vi "Process.vi"(8 "error in":errorcluster, 11 "Instrument":refnum<class "Instrument.lvclass">) -> (0 "error out":errorcluster, 3 "Instrument out":refnum<class "Instrument.lvclass">)   [LabVIEW 2019, in "Instrument.lvclass"]
doc: "---------------------------------------------------------------\nJKI State Machine Objects™\nhttp://jki.net/state-machine-objects/\nCopyright (C) 2005-2015, JKI <info@jki.net>\nALL RIGHTS RESERVED"
uses:
  Instrument.lvclass
  C:/Program Files (x86)/National Instruments/LabVIEW 2019/vi.lib/JKI/JKI SMO/SMO/SMO.lvclass
  Typedefs/PrivateEvents--Instrument.DataToLog.ctl
  Instrument.lvclass/Instrument.ctl
  <userlib>/LevyLab/RemoteControl/Typedefs/Message--Cluster.ctl
  Typedefs/PrivateEvents--LogTime.ctl
  <vilib>/JKI/JKI SMO/SMO/SMO.lvclass/SMO.ctl
  <vilib>/JKI/JKI SMO/SMO/Private/ReftoDVR--SMO.vi
  <userlib>/LevyLab/RemoteControl/RemoteControl.lvclass
  <userlib>/LevyLab/Logger.Error/Logger.Error.lvclass
  <userlib>/LevyLab/Logger.PGSQL/Logger.PGSQL.lvclass
  <vilib>/JKI/JKI SMO/SMO/SMO.lvclass
  C:/Program Files (x86)/National Instruments/LabVIEW 2019/user.lib/LevyLab/Logger/Logger.lvclass
  <userlib>/LevyLab/Configuration/Debug.lvlib
panel:
  out "State History":string
  out "Name":string
  out "Command":string
  # "1. Receives & processes commands from RemoteControl process\n2. Logs instrument settings to PGSQL using Logger process"
  # "INSTRUMENT"
  # "INSTRUMENT"
  # "For instructions on how to use the JKI State Machine Objects, examples and video tutorials, visit:\nhttp://jki.net/state-machine-objects/\n\nJKI State Machine Objects™\nhttp://jki.net/state-machine-objects/\nCopyright (C) 2005-2015, JKI <info@jki.net>\nALL RIGHTS RESERVED"
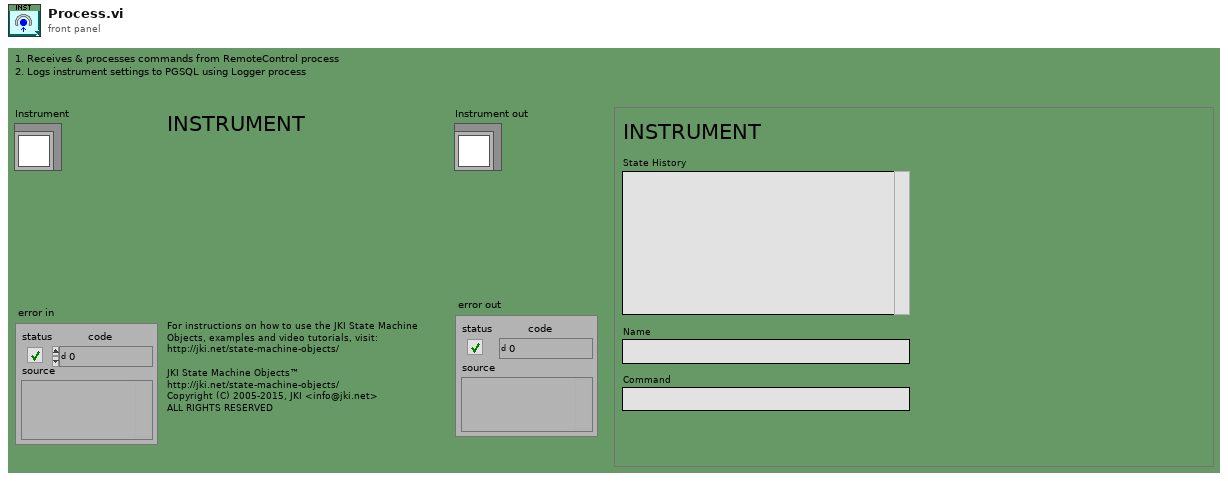
[diagram p1: front panel]
types:
  T1 = typedef "Instrument.lvclass/PrivateEvents--Instrument.DataToLog.ctl" = cluster{"path":string, "Data":variant}
  T2 = enum32{"invalid app kind", "Development System", "Run Time System", "Student Edition", "Embedded LabVIEW", "Evaluation", "Custom"}
  T3 = enum32{"Invalid", "Standard", "Closed", "Hidden", "Minimized", "Maximized"}
  T4 = typedef "RemoteControl.lvclass/Message--Cluster.ctl" = cluster{"Command":string, "Data":variant, "ID":string}
  T5 = typedef "Instrument.lvclass/PrivateEvents--LogTime.ctl" = u32
  T6 = typedef "Instrument.lvclass/Dependencies--Cluster.ctl" = cluster{"API":refnum<class "API.lvclass">, "Configuration":refnum<class "Configuration.lvclass">, "HAL":refnum<class "HAL.lvclass">, "DB-Logger":refnum<class "Logger.PGSQL.lvclass">, "Error-Logger":refnum<class "Logger.Error.lvclass">, "Remote-Control":refnum<class "RemoteControl.lvclass">}
  T7 = typedef "Debug.lvlib/Attribute.Debug.lvclass/DebugBehavior.ctl" = enum16{"Normal", "Debug"}
  T8 = cluster{"Core":cluster{"Current VI Reference":refnum<vi>, "Close Panel on Exit?":bool, "Last Error":cluster{"error":errorcluster, "previous state":string, "remaining states":string}, "Shutdown?":bool}, "SelfRef":refnum<class "Instrument.lvclass">, "Dependencies":T6, "Message":T4, "LogTime":T5, "Behavior":T7}
  T9 = typedef "SMO.lvclass/SMOState --Enum.ctl" = enum16{"unknown", "Created", "Started", "Stopped"}
  T10 = cluster{"Current VI Reference":refnum<vi>, "Close Panel on Exit?":bool, "Last Error":cluster{"error":errorcluster, "previous state":string, "remaining states":string}, "Shutdown?":bool}
  T11 = typedef "SMO.lvclass/Protected Events.ctl" = cluster{"StopProcesses":refnum<user-event>, "AbortProcesses":refnum<user-event>, "Config Changed":refnum<user-event>, "Dependency":refnum<user-event>}
  T12 = typedef "Instrument.lvclass/PrivateEvents--Cluster.ctl" = cluster{"MessageToProcess":refnum<user-event>, "LogData":refnum<user-event>, "LogTime":refnum<user-event>}
  T13 = typedef "RemoteControl.lvclass/PublicEvents--Cluster.ctl" = cluster{"SendMessageFromProcess":refnum<user-event>}
  T14 = typedef "SMO.lvclass/Public Events.ctl" = cluster{"Error":refnum<user-event>, "State":refnum<user-event>, "Reserve State":refnum<user-event>}
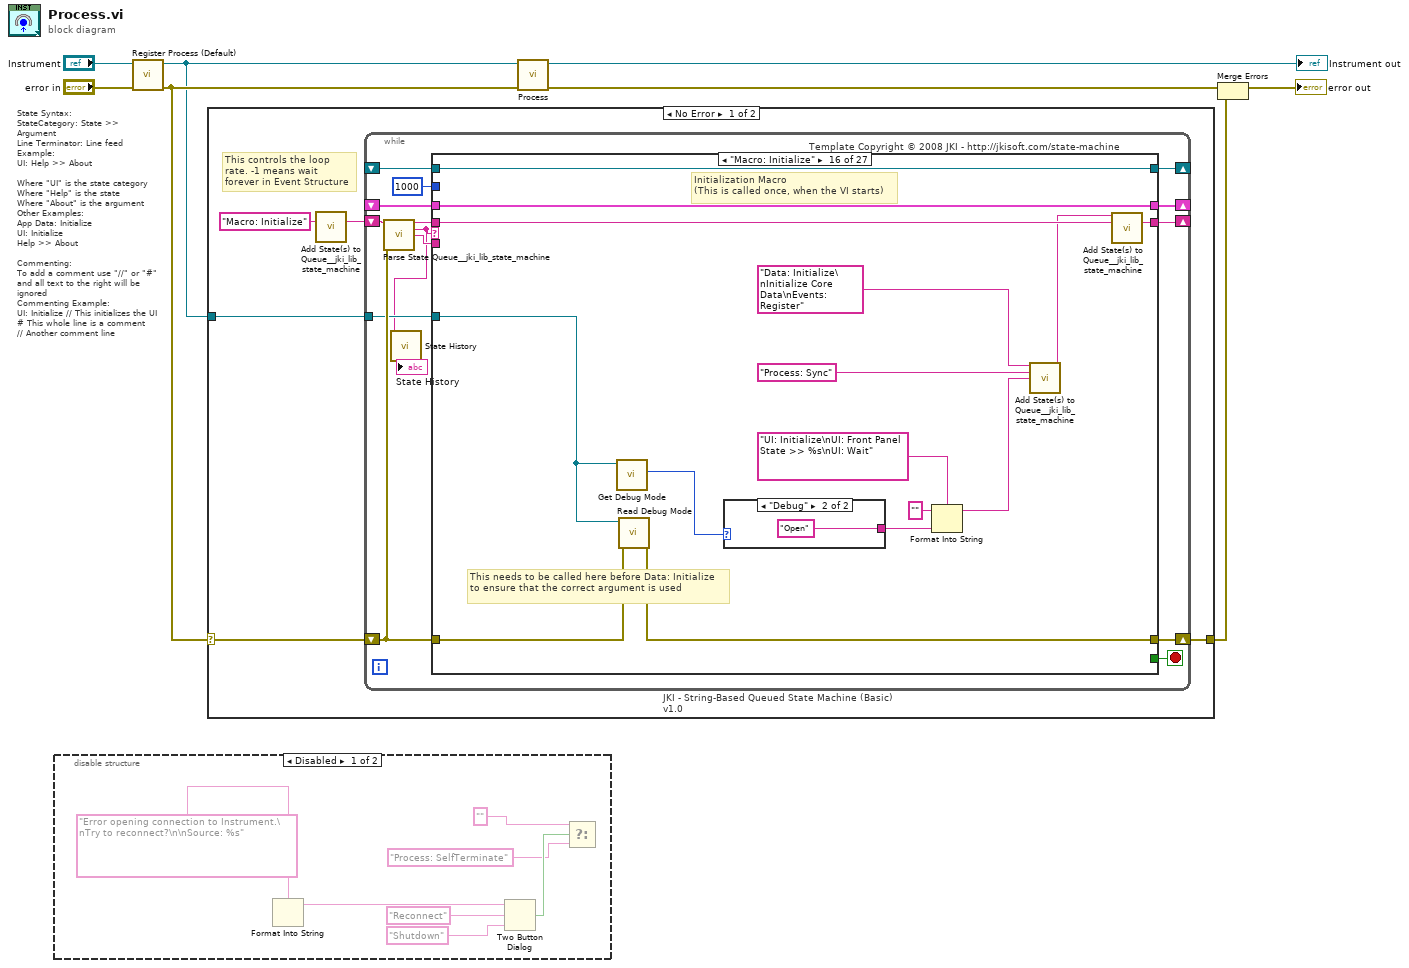
[diagram p0: block diagram]
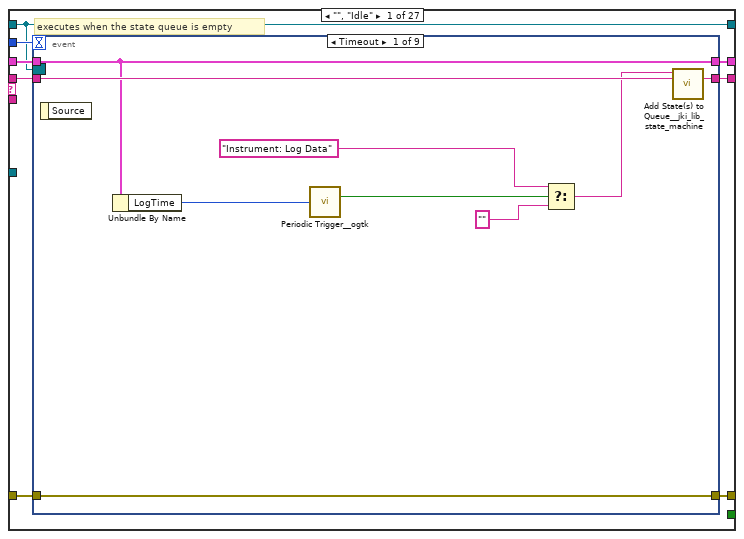
[diagram p3: hidden frame]
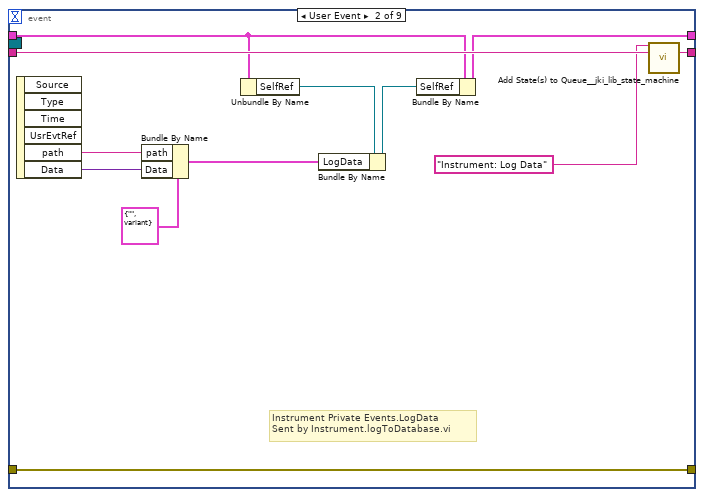
[diagram p4: hidden frame]
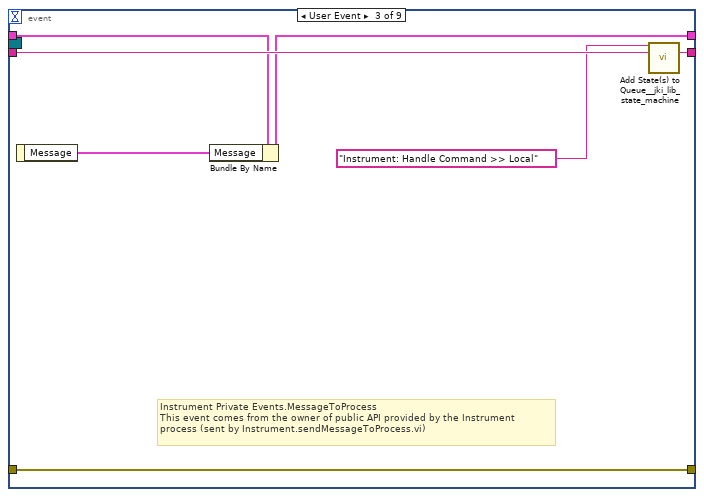
[diagram p5: hidden frame]
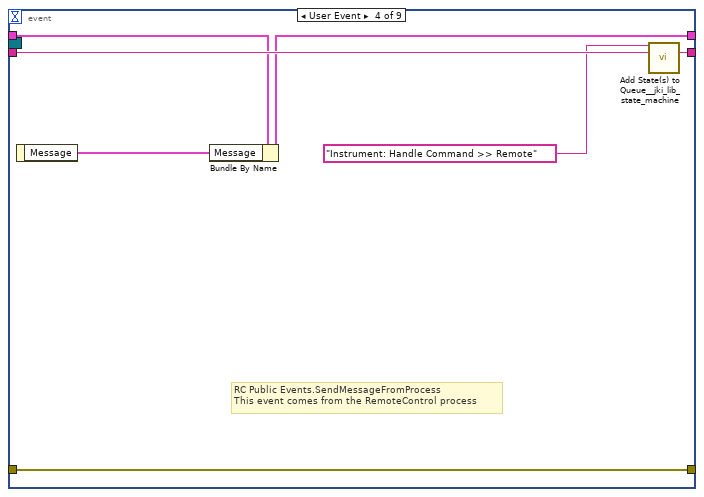
[diagram p6: hidden frame]
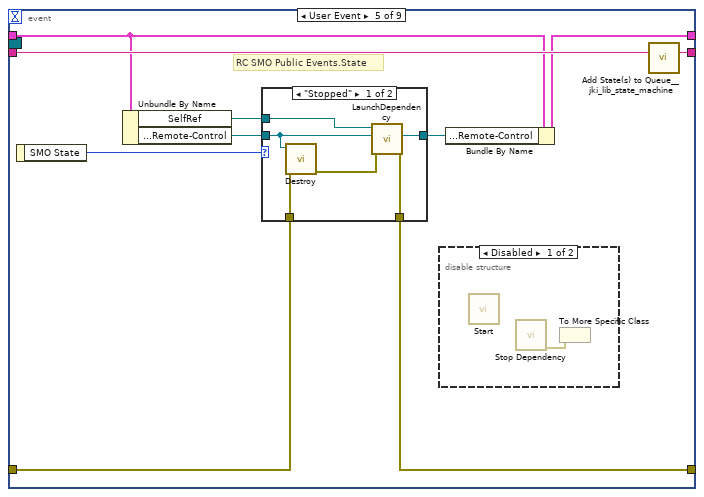
[diagram p7: hidden frame]
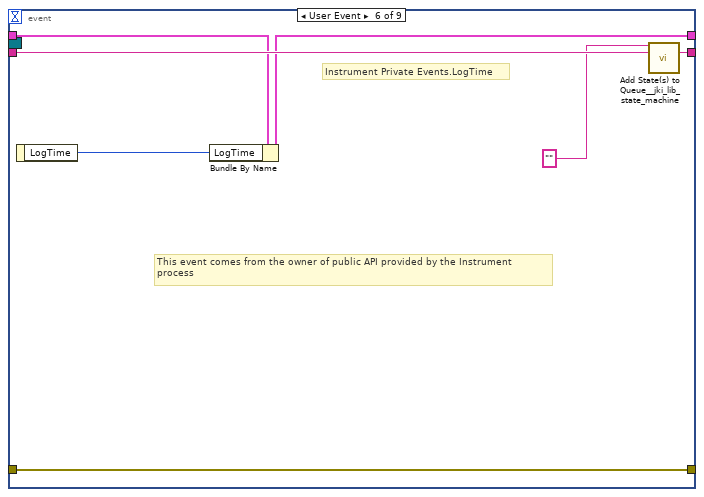
[diagram p10: hidden frame]
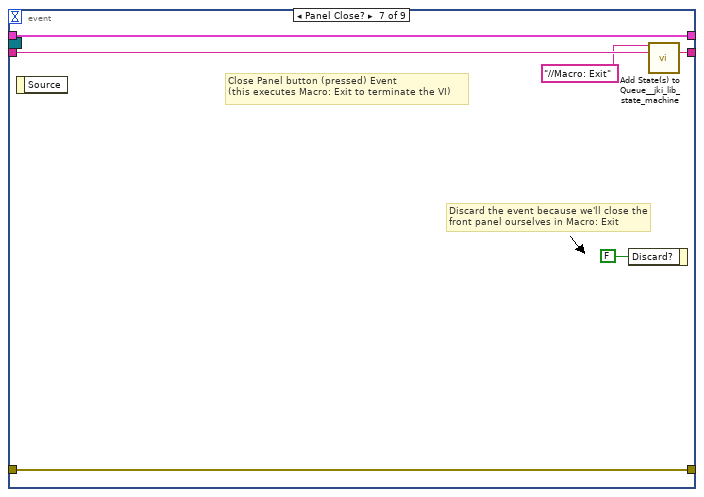
[diagram p11: hidden frame]
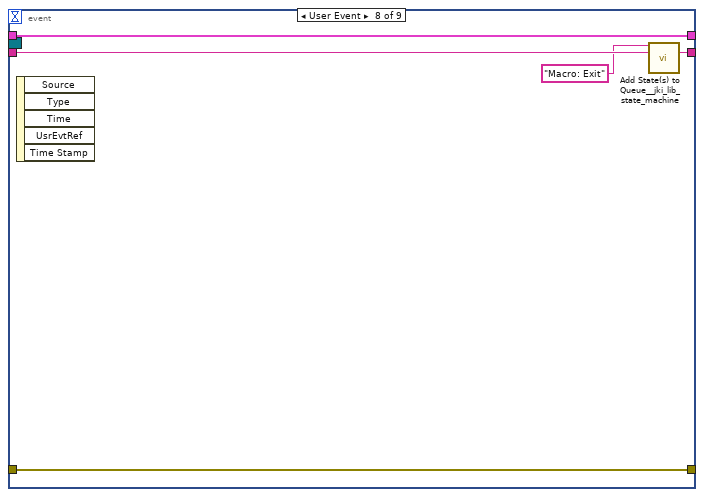
[diagram p12: hidden frame]
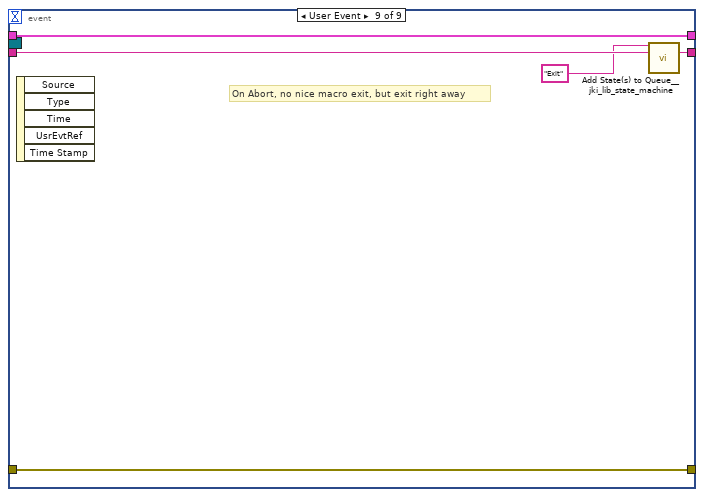
[diagram p13: hidden frame]
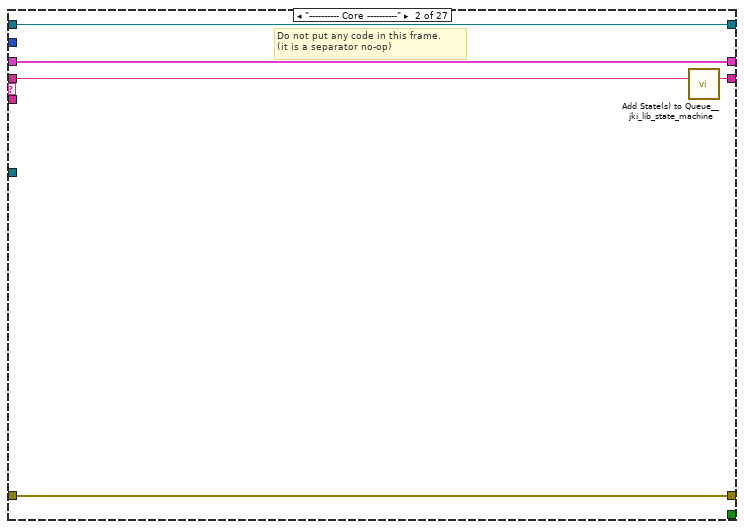
[diagram p14: hidden frame]
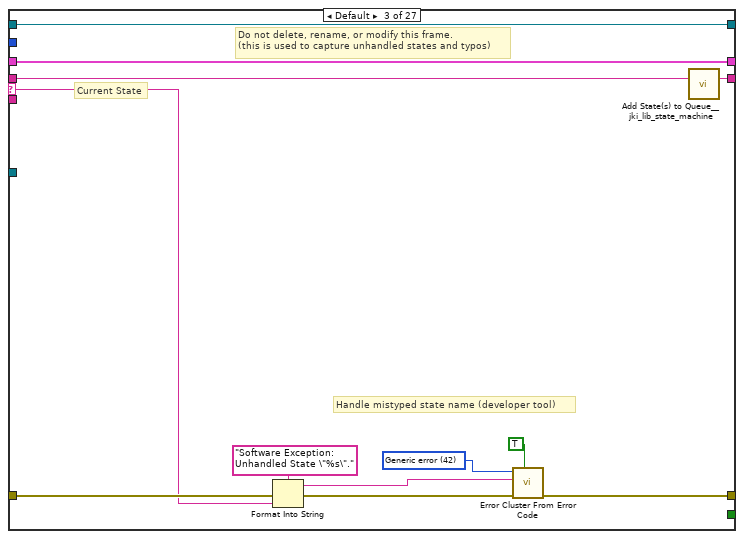
[diagram p15: hidden frame]
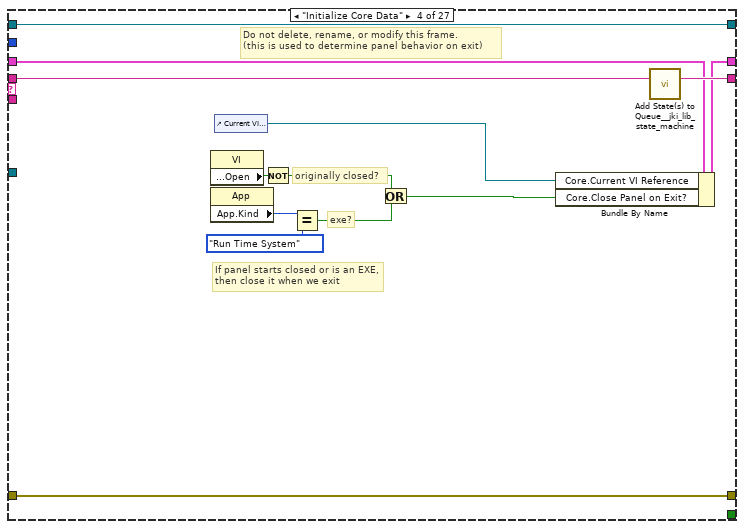
[diagram p16: hidden frame]
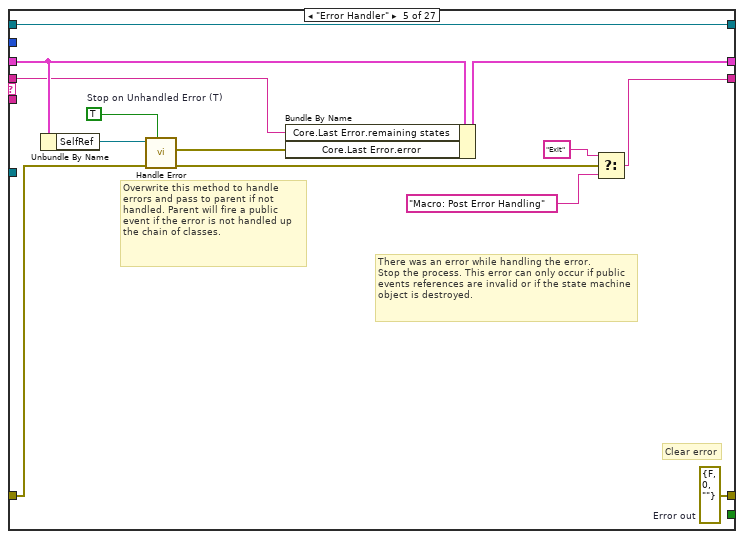
[diagram p17: hidden frame]
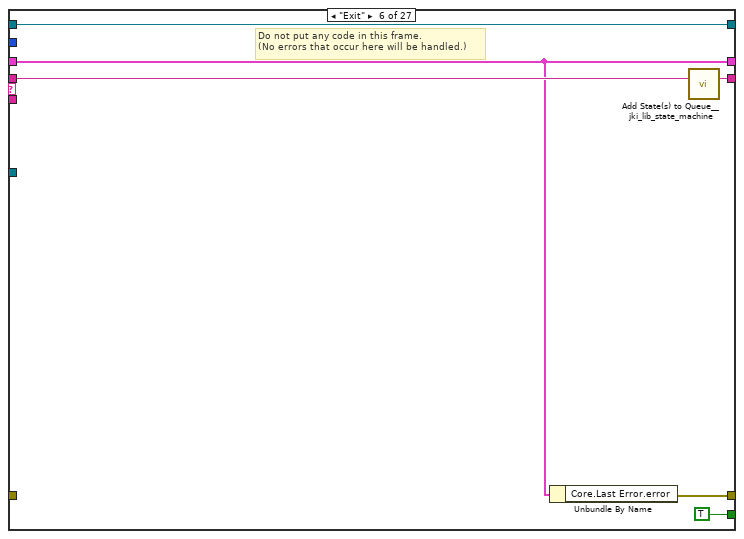
[diagram p18: hidden frame]
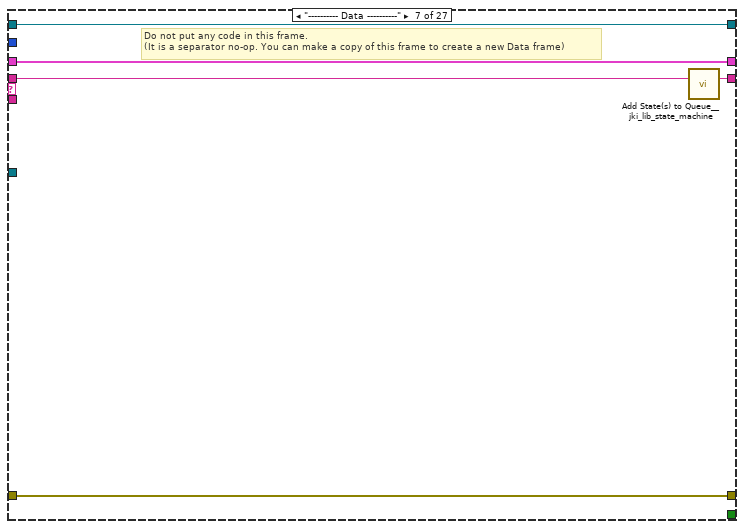
[diagram p19: hidden frame]
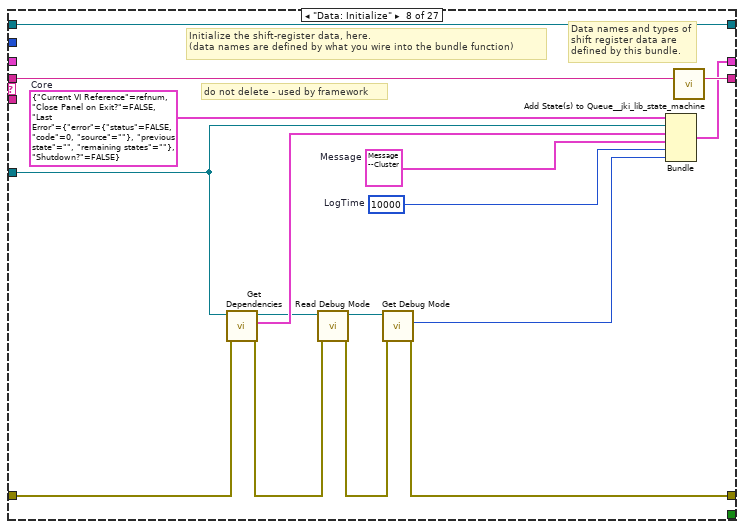
[diagram p20: hidden frame]
diagram:
  # "State Syntax:\nStateCategory: State >> Argument\nLine Terminator: Line feed\nExample:\nUI: Help >> About\n\nWhere \"UI\" is the state category\nWhere \"Help\" is the state\nWhere \"About\" is the argument\nOther Examples:\nApp Data: Initialize\nUI: Initialize\nHelp >> About\n\nCommenting:\nTo add a comment use \"//\" or \"#\" and all text to the right will be ignored\nCommenting Example:\nUI: Initialize // This initializes the UI\n# This whole line is a comment\n// Another comment line"
  n1 = disable-structure shown="Disabled" {
    frame Disabled {
      n2 = Format Into String(format string="Error opening connection to Instrument.\nTry to reconnect?\n\nSource: %s" ("message")) -> (resulting string=w9:string)  [unwired: 3 in, 1 out]
      n3 = Two Button Dialog(message=w9, 1:"Shutdown" ("F button name (\"Cancel\")"), 2:"Reconnect" ("T button name (\"OK\")")) -> (T button?=w13:bool)
      n4 = Select(t="" ("States to Execute"), s=w13, f="Process: SelfTerminate" ("States to Execute")) -> ()  [unwired: 1 out]
    }
    frame Enabled {
    }
  }
  n5 = call <vilib>:"Register Process (Default).vi"("error in (no error)"="error in", "SMO"="Instrument") -> ("error out"=w5:errorcluster, "SelfRef"=w4:refnum<class "Instrument.lvclass">)  [unwired: 8 in]
  n6 = case shown="No Error" w5 {
    selector: w5 -> [w17 w462]
    tunnel: w4 -> [w18 _]
    tunnel: [w16 w462] -> w1
    frame No Error {
      # "This controls the loop rate. -1 means wait forever in Event Structure"
      n7 = call <vilib>:"Add State(s) to Queue__jki_lib_state_machine.vi"("State(s) in (\"\")"="Macro: Initialize") -> ("States Out"=w20:string)  [unwired: 14 in]
      n8 = while "JKI - String-Based Queued State Machine (Basic) v1.0" {
        shift-right: [w29] -> _
        shift-left: _ -> [w28]
        shift-right: [w32] -> w16
        shift-left: w17 -> [w26]
        shift-right: [w31] -> _
        shift-left: w20 -> [w33]
        tunnel: w18 -> [w23]
        shift-right: [w25] -> _
        shift-left: _ -> [w24]
        stop <- w30 stop-if-true
        # "Template Copyright © 2008 JKI - http://jkisoft.com/state-machine"
        n9 = call <vilib>:"Parse State Queue__jki_lib_state_machine.vi"("State Queue"=w33, "Error In (no error)"=w26) -> ("Remaining States"=w35:string, "Current State"=w22:string, "Arguments"=w34:string)  [unwired: 11 in]
        n10 = call "State History.vi"("Current State"=w22) -> ("History"=→"State History":string)  [unwired: 10 in]
        n11 = case shown="\"Macro: Initialize\"" w22 {
          selector: w22 -> [_ _ w127 _ _ _ _ _ _ _ _ _ _ _ _ _ _ _ _ _ _ _ _ _ _ _ _]
          tunnel: w35 -> [w43 w125 w131 w150 w152 w169 w174 w190 w197 w202 w212 w219 w235 w270 w277 w292 w311 w317 w334 w345 w354 w359 w390 w396 w401 w424 w461]
          tunnel: w34 -> [_ _ _ _ _ _ _ _ _ _ _ w213 w229 _ _ _ _ _ _ _ _ _ _ _ _ w404 _]
          tunnel: w28 -> [w41 w122 w129 w141 w161 w165 w171 _ w192 w199 w209 w217 w231 w265 w274 w286 w303 w320 w331 w342 w349 w356 w388 w394 w399 w417 w455]
          tunnel: [w40 w123 w133 w147 w162 w164 w172 w175 w193 w200 w203 w214 w232 w266 w275 w284 w309 w324 w332 w336 w346 w357 w386 w392 w397 w409 w456] -> w32
          tunnel: w26 -> [w39 w123 w132 w147 w153 _ w172 w180 w194 w200 w206 w215 w233 w267 w275 w285 w309 w324 w332 w337 w347 w357 w384 w392 w397 w420 w457]
          tunnel: [w42 w124 w130 w149 w157 w168 w173 w189 w196 w201 w211 w218 w234 w269 w276 w291 w310 w318 w333 w344 w353 w358 w389 w395 w400 w423 w460] -> w31
          tunnel: [_ _ _ _ _ TRUE _ _ _ _ _ _ _ _ _ _ _ _ _ _ _ _ _ _ _ _ _] -> w30
          tunnel: [w38 w122 w129 w148 w160 w165 w171 w184 w192 w199 w209 w217 w231 w265 w274 w286 w303 w321 w331 w342 w348 w356 w388 w394 w399 w416 w455] -> w29
          tunnel: 1000 ("Timeout") -> [w37 _ _ _ _ _ _ _ _ _ _ _ _ _ _ _ _ _ _ _ _ _ _ _ _ _ _]
          tunnel: [w36 w121 w126 w138 w163 w166 w170 w188 w191 w198 w210 w216 w228 w268 w273 w290 w304 w325 w330 w343 w352 w355 w387 w393 w398 w422 w459] -> w25
          tunnel: w24 -> [w36 w121 w126 w138 w163 w166 w170 w188 w191 w198 w210 w216 w228 w268 w273 w290 w304 w325 w330 w343 w352 w355 _ w393 w398 w422 w459]
          tunnel: w23 -> [_ _ _ _ _ _ _ w182 _ _ _ _ _ _ _ w280 _ _ _ _ _ _ _ _ _ _ _]
          frame "", "Idle" {
            # "executes when the state queue is empty"
            n12 = event shown="[0] Timeout" {
              selector: w36 -> [_ _ _ _ _ _ _ _ _]
              dyn-events: _ -> [_ _ _ _ _ _ _ _ _]
              timeout: w37 -> [_ _ _ _ _ _ _ _ _]
              tunnel: w43 -> [w52 w64 w71 w78 w88 w104 w110 w115 w120]
              tunnel: [w51 w63 w70 w77 w87 w103 w109 w114 w119] -> w42
              tunnel: w41 -> [w45 w55 w68 w75 w84 w101 w107 w112 w117]
              tunnel: [w50 w62 w69 w76 w81 w102 w108 w113 w118] -> w40
              tunnel: w39 -> [w50 w62 w69 w76 w82 w102 w108 w113 w118]
              tunnel: [w45 w53 w67 w74 w83 w100 w107 w112 w117] -> w38
              event Timeout {
                n13 = event-data() -> ()  [unwired: 1 in, 1 out]
                n14 = Unbundle By Name(w45) -> ("LogTime"=w44:T5)
                n15 = call <userlib>:"Periodic Trigger__ogtk.vi"("time (ms)"=w44) -> ("Triggered"=w48:bool)  [unwired: 12 in, 2 out]
                n16 = Select(t="Instrument: Log Data" ("State(s) in Front (\"\")"), s=w48, f="") -> (s? t:f=w49:string)
                n17 = call <vilib>:"Add State(s) to Queue__jki_lib_state_machine.vi"("State(s) in Front (\"\")"=w49, "State(s) in (\"\")"=w52) -> ("States Out"=w51:string)  [unwired: 13 in]
              }
              event User Event {
                # "Instrument Private Events.LogData\nSent by Instrument.logToDatabase.vi"
                n18 = event-data() -> ("path"=w58:string, "Data"=w59:variant)  [unwired: 1 in, 4 out]
                n19 = Bundle By Name(cluster=T1 {"path"="", "Data"=variant} ("Log Data"), "path"=w58, "Data"=w59) -> (w57:T1)
                n20 = Unbundle By Name(w55) -> ("SelfRef"=w56:refnum<class "Instrument.lvclass">)
                n21 = Bundle By Name(cluster=w56, "LogData"=w57) -> (w54:refnum<class "Instrument.lvclass">)
                n22 = Bundle By Name(cluster=w55, "SelfRef"=w54) -> (w53:T8)
                n23 = call <vilib>:"Add State(s) to Queue__jki_lib_state_machine.vi"("State(s) in Front (\"\")"="Instrument: Log Data" ("State(s) in Front (\"\")"), "State(s) in (\"\")"=w64) -> ("States Out"=w63:string)  [unwired: 13 in]
              }
              event User Event {
                # "Instrument Private Events.MessageToProcess\nThis event comes from the owner of public API provided by the Instrument\nprocess (sent by Instrument.sendMessageToProcess.vi)"
                n24 = event-data() -> ("Message"=w66:T4)  [unwired: 1 in]
                n25 = Bundle By Name(cluster=w68, "Message"=w66) -> (w67:T8)
                n26 = call <vilib>:"Add State(s) to Queue__jki_lib_state_machine.vi"("State(s) in Front (\"\")"="Instrument: Handle Command >> Local" ("State(s) in Front (\"\")"), "State(s) in (\"\")"=w71) -> ("States Out"=w70:string)  [unwired: 13 in]
              }
              event User Event {
                # "RC Public Events.SendMessageFromProcess\nThis event comes from the RemoteControl process"
                n27 = event-data() -> ("Message"=w73:T4)  [unwired: 1 in]
                n28 = Bundle By Name(cluster=w75, "Message"=w73) -> (w74:T8)
                n29 = call <vilib>:"Add State(s) to Queue__jki_lib_state_machine.vi"("State(s) in Front (\"\")"="Instrument: Handle Command >> Remote" ("State(s) in Front (\"\")"), "State(s) in (\"\")"=w78) -> ("States Out"=w77:string)  [unwired: 13 in]
              }
              event User Event {
                # "RC SMO Public Events.State"
                n30 = event-data() -> ("SMO State"=w79:T9)  [unwired: 1 in]
                n31 = Unbundle By Name(w84) -> ("SelfRef"=w80:refnum<class "Instrument.lvclass">, "Dependencies.Remote-Control"=w86:refnum<class "RemoteControl.lvclass">)
                n32 = case shown="\"Stopped\"" w79 {
                  tunnel: w86 -> [w90 w97]
                  tunnel: [w95 w97] -> w85
                  tunnel: w82 -> [w92 w96]
                  tunnel: [w94 w96] -> w81
                  tunnel: w80 -> [w93 _]
                  frame "Stopped" {
                    n33 = call <vilib>:"Destroy.vi"("error in (no error)"=w92, "SMO"=w90) -> ("error out"=w91:errorcluster)  [unwired: 9 in]
                    n34 = call <vilib>:"LaunchDependency.vi"("error in (no error)"=w91, "Dependency Type"=w90, "SMO in"=w93) -> ("error out"=w94:errorcluster, "Dependency Reference"=w95:refnum<class "RemoteControl.lvclass">)  [unwired: 5 in, 2 out]
                  }
                  frame Default {
                  }
                }
                n35 = disable-structure shown="Disabled" {
                  frame Disabled {
                    n36 = call <vilib>:"Start.vi"() -> ()  [unwired: 10 in, 2 out]
                    n37 = call <vilib>:"Stop Dependency.vi"() -> ("error out"=w89:errorcluster)  [unwired: 9 in, 2 out]
                    n38 = To More Specific Class(error in=w89) -> ()  [unwired: 2 in, 2 out]
                  }
                  frame Enabled {
                  }
                }
                n39 = Bundle By Name(cluster=w84, "Dependencies.Remote-Control"=w85) -> (w83:T8)
                n40 = call <vilib>:"Add State(s) to Queue__jki_lib_state_machine.vi"("State(s) in (\"\")"=w88) -> ("States Out"=w87:string)  [unwired: 14 in]
              }
              event User Event {
                # "Instrument Private Events.LogTime"
                # "This event comes from the owner of public API provided by the Instrument\nprocess"
                n41 = event-data() -> ("LogTime"=w99:T5)  [unwired: 1 in]
                n42 = Bundle By Name(cluster=w101, "LogTime"=w99) -> (w100:T8)
                n43 = call <vilib>:"Add State(s) to Queue__jki_lib_state_machine.vi"("State(s) in Front (\"\")"="" ("State(s) in Front (\"\")"), "State(s) in (\"\")"=w104) -> ("States Out"=w103:string)  [unwired: 13 in]
              }
              event Panel Close? {
                # "Discard the event because we'll close the front panel ourselves in Macro: Exit"
                # "Close Panel button (pressed) Event\n(this executes Macro: Exit to terminate the VI)"
                n44 = event-data() -> ()  [unwired: 1 in, 1 out]
                n45 = event-data("Discard?"=FALSE) -> ()  [unwired: 1 in, 1 out]
                n46 = call <vilib>:"Add State(s) to Queue__jki_lib_state_machine.vi"("State(s) in Front (\"\")"="//Macro: Exit", "State(s) in (\"\")"=w110) -> ("States Out"=w109:string)  [unwired: 13 in]
              }
              event User Event {
                n47 = event-data() -> ()  [unwired: 1 in, 5 out]
                n48 = call <vilib>:"Add State(s) to Queue__jki_lib_state_machine.vi"("State(s) in Front (\"\")"="Macro: Exit", "State(s) in (\"\")"=w115) -> ("States Out"=w114:string)  [unwired: 13 in]
              }
              event User Event {
                # "On Abort, no nice macro exit, but exit right away"
                n49 = event-data() -> ()  [unwired: 1 in, 5 out]
                n50 = call <vilib>:"Add State(s) to Queue__jki_lib_state_machine.vi"("State(s) in Front (\"\")"="Exit", "State(s) in (\"\")"=w120) -> ("States Out"=w119:string)  [unwired: 13 in]
              }
            }
          }
          frame "---------- Core ----------" {
            # "Do not put any code in this frame.\n(it is a separator no-op)"
            n51 = call <vilib>:"Add State(s) to Queue__jki_lib_state_machine.vi"("State(s) in (\"\")"=w125) -> ("States Out"=w124:string)  [unwired: 14 in]
          }
          frame Default {
            w136 = 42 items=["No error", "Argument error", "Memory is full", "Out of zone", "End of file", "File already open", "Generic file I/O error", "File not found", "File permission error", "Disk is full", "Duplicate path", "Too many files open", "System feature not enabled", "Resource file not found", "Cannot add resource", "Resource not found", "Image not found", "Image memory error", "Pen does not exist", "Config type invalid", "Config token not found", "Config parse error", "Config memory error", "Bad external code format", "Bad external code offset", "External code not present", "Null window", "Destroy window error", "Null menu", "Print aborted", "Bad print record", "Print driver error", "Windows error during printing", "Memory error during printing", "Print dialog error", "Generic print error", "Invalid device refnum", "Device not found", "Device parameter error", "Device unit error", "Cannot open device", "Device call aborted", "Generic error", "Cancelled by user", "Object ID too low", "Object ID too high", "Object not in heap", "Unknown heap", "Unknown object (invalid DefProc)", "Unknown object (DefProc not in table)", "Message out of range", "Invalid (null) method", "Unknown message", "Manager call not supported", "Bad address", "Network operation in progress", "Network operation timed out", "Connection is busy", "Network attribute not supported", "Network error", "Address in use", "System out of memory", "Connection aborted", "Connection refused", "Not connected", "Already connected", "Connection closed", "Initialization error (interapplication manager)", "Bad occurrence", "Wait on unbound occurrence handler", "Occurrence queue overflow", "Datalog type conflict", "Unused", "Unrecognized type (interapplication manager)", "Memory corrupt", "Failed to make temporary DLL", "Old CIN version", "Drag socket not found", "Failed to load drop-object", "Failed to register OLE object", "Failed to release OLE object", "Format specifier type mismatch", "Unknown format specifier", "Too few format specifiers", "Too many format specifiers", "Scan failed", "Newer CIN version", "Error converting to variant", "Runtime menu error", "Password tampered", "Variant attribute not found", "Incompatible variant data type", "Event data is not available", "Event Store is not present", "Occurrence is not found", "Event Queue is not created", "Event info is not available", "Refnum passed is NULL", "Error retrieving Class GUID", "Error retrieving CoClass GUID", "Error retrieving TypeLib GUID.", "Bad built application magic bytes.", "Specific driver is different from the specific driver associated with the Logical Name.", "There is no session opened to the class driver.", "Max Error", "MAX - Error with config objects", "MAX - Error loading configuration", "MAX - Group not supported"]
            # "Current State"
            # "Do not delete, rename, or modify this frame.\n(this is used to capture unhandled states and typos)"
            # "Handle mistyped state name (developer tool)"
            n52 = Format Into String(format string="Software Exception: Unhandled State \"%s\"." ("message"), error in=w132, w127) -> (resulting string=w135:string, error out=w134:errorcluster)  [unwired: 1 in]
            n53 = call <vilib>:"Error Cluster From Error Code.vi"("show call chain? (False)"=TRUE, "error in (no error)"=w134, "error message (\"\")"=w135, "error code (0)"=w136) -> ("error out"=w133:errorcluster)  [unwired: 5 in]
            n54 = call <vilib>:"Add State(s) to Queue__jki_lib_state_machine.vi"("State(s) in (\"\")"=w131) -> ("States Out"=w130:string)  [unwired: 14 in]
          }
          frame "Initialize Core Data" {
            # "Do not delete, rename, or modify this frame.\n(this is used to determine panel behavior on exit)"
            # "originally closed?"
            # "exe?"
            # "If panel starts closed or is an EXE, then close it when we exit"
            n55 = property class="VI"() -> ("Front Panel.Open"=w146:bool)  [unwired: 2 in, 2 out]
            n56 = property class="App"() -> ("App.Kind"=w145:T2)  [unwired: 2 in, 2 out]
            n57 = control-ref of="Current VI Reference"() -> (w139:refnum<vi>)
            n58 = Not(x=w146) -> (.not. x?=w143:bool)
            n59 = Equal?(x=w145, y=T2."Run Time System" ("Application:Kind")) -> (x = y?=w142:bool)
            n60 = Or(x=w143, y=w142) -> (x .or. y?=w140:bool)
            n61 = Bundle By Name(cluster=w141, "Core.Current VI Reference"=w139, "Core.Close Panel on Exit?"=w140) -> (w148:T8)
            n62 = call <vilib>:"Add State(s) to Queue__jki_lib_state_machine.vi"("State(s) in (\"\")"=w150) -> ("States Out"=w149:string)  [unwired: 14 in]
          }
          frame "Error Handler" {
            w158 = TRUE  # Stop on Unhandled Error (T)
            w162 = errorcluster {"status"=FALSE, "code"=0, "source"=""}  # Error out
            # "Clear error"
            # "There was an error while handling the error.\nStop the process. This error can only occur if public events references are invalid or if the state machine object is destroyed."
            # "Overwrite this method to handle errors and pass to parent if not handled. Parent will fire a public event if the error is not handled up the chain of classes."
            n63 = Unbundle By Name(w161) -> ("SelfRef"=w154:refnum<class "Instrument.lvclass">)
            n64 = call-dynamic "Handle Error.vi"("Stop on Unhandled Error (T)"=w158, "error in"=w153, "SMO"=w154) -> ("handling error"=w155:errorcluster, "Unhandled error"=w156:errorcluster)  [unwired: 6 in, 1 out]
            n65 = Bundle By Name(cluster=w161, "Core.Last Error.remaining states"=w152, "Core.Last Error.error"=w156) -> (w160:T8)
            n66 = Select(t="Exit", s=w155, f="Macro: Post Error Handling" ("State")) -> (s? t:f=w157:string)
          }
          frame "Exit" {
            # "Do not put any code in this frame.\n(No errors that occur here will be handled.)"
            n67 = Unbundle By Name(w165) -> ("Core.Last Error.error"=w164:errorcluster)
            n68 = call <vilib>:"Add State(s) to Queue__jki_lib_state_machine.vi"("State(s) in (\"\")"=w169) -> ("States Out"=w168:string)  [unwired: 14 in]
          }
          frame "---------- Data ----------" {
            # "Do not put any code in this frame.\n(It is a separator no-op. You can make a copy of this frame to create a new Data frame)"
            n69 = call <vilib>:"Add State(s) to Queue__jki_lib_state_machine.vi"("State(s) in (\"\")"=w174) -> ("States Out"=w173:string)  [unwired: 14 in]
          }
          frame "Data: Initialize" {
            w185 = T5 10000  # LogTime
            w186 = T4 {"Command"="", "Data"=variant(string ""), "ID"=""}  # Message
            w187 = T10 {"Current VI Reference"=refnum, "Close Panel on Exit?"=FALSE, "Last Error"={"error"={"status"=FALSE, "code"=0, "source"=""}, "previous state"="", "remaining states"=""}, "Shutdown?"=FALSE}  # Core
            # "do not delete - used by framework"
            # "Data names and types of shift register data are defined by this bundle."
            # "Initialize the shift-register data, here.\n(data names are defined by what you wire into the bundle function)"
            n70 = call "Get Dependencies.vi"("error in (no error)"=w180, "Instrument in"=w182) -> ("error out"=w181:errorcluster, "Dependencies"=w183:T6, "Instrument out"=w178:refnum<class "Instrument.lvclass">)  [unwired: 7 in]
            n71 = call-dynamic "Read Debug Mode.vi"("error in (no error)"=w181, "Instrument in"=w178) -> ("error out"=w176:errorcluster, "Instrument out"=w177:refnum<class "Instrument.lvclass">)  [unwired: 7 in, 1 out]
            n72 = call <userlib>:"Get Debug Mode.vi"("error in (no error)"=w176, "SMO"=w177) -> ("error out"=w175:errorcluster, "Behavior"=w179:T7)  [unwired: 7 in, 1 out]
            n73 = Bundle("Core"=w187, "SelfRef"=w182, "Dependencies"=w183, "Message"=w186, "LogTime"=w185, "Behavior"=w179) -> (w184:T8)  [unwired: 1 in]
            n74 = call <vilib>:"Add State(s) to Queue__jki_lib_state_machine.vi"("State(s) in (\"\")"=w190) -> ("States Out"=w189:string)  [unwired: 14 in]
          }
          frame "Data: Cleanup" {
            # "Cleanup any data and references, here.\n(this is called automatically, by the Macro: Exit)"
            n75 = Unbundle By Name(w192) -> ("Core.Current VI Reference"=w195:refnum<vi>)
            n76 = Close Reference(reference=w195, error in (no error)=w194) -> (error out=w193:errorcluster)
            n77 = call <vilib>:"Add State(s) to Queue__jki_lib_state_machine.vi"("State(s) in (\"\")"=w197) -> ("States Out"=w196:string)  [unwired: 14 in]
          }
          frame "---------- UI ----------" {
            # "Do not put any code in this frame.\n(It is a separator no-op. You can make a copy of this frame to create a new UI frame)"
            n78 = call <vilib>:"Add State(s) to Queue__jki_lib_state_machine.vi"("State(s) in (\"\")"=w202) -> ("States Out"=w201:string)  [unwired: 14 in]
          }
          frame "UI: Initialize" {
            # "Initialize the User Interface, here.\n(this is called automatically, by the Macro: Init)"
            n79 = Unbundle By Name(w209) -> ("SelfRef"=w208:refnum<class "Instrument.lvclass">)
            n80 = call <vilib>:"GetName.vi"("error in (no error)"=w206, "SMO"=w208) -> ("error out"=w204:errorcluster, "Name"=→"Name":string)  [unwired: 6 in, 2 out]
            n81 = call <userlib>:"Fit VI window to Largest Dec__ogtk.vi"("error in (no error)"=w204, "border spacing (2 px)"=0) -> ("error out"=w203:errorcluster)  [unwired: 4 in, 1 out]
            n82 = call <vilib>:"Add State(s) to Queue__jki_lib_state_machine.vi"("State(s) in (\"\")"=w212) -> ("States Out"=w211:string)  [unwired: 14 in]
          }
          frame "UI: Cursor Set" {
            # "Argument"
            # "Initialize the User Interface, here.\n(this is called automatically, by the Macro: Init)"
            n83 = disable-structure shown="Default" {
              disable-tunnel: w215 -> [w220 w223]
              disable-tunnel: [w220 w222] -> w214
              disable-tunnel: w213 -> [_ w221]
              frame condition #0 {
              }
              frame condition #1 (active) {
                n84 = case shown="\"Busy\"" w221 {
                  tunnel: w223 -> [w225 w227]
                  tunnel: [w224 w226] -> w222
                  frame "Idle", Default {
                    n85 = call <vilib>:"Unset Busy.vi"("error in (no error)"=w225) -> ("error out"=w224:errorcluster)  [unwired: 10 in]
                  }
                  frame "Busy" {
                    n86 = call <vilib>:"Set Busy.vi"("error in (no error)"=w227) -> ("error out"=w226:errorcluster)  [unwired: 9 in, 1 out]
                  }
                }
              }
            }
            n87 = call <vilib>:"Add State(s) to Queue__jki_lib_state_machine.vi"("State(s) in (\"\")"=w219) -> ("States Out"=w218:string)  [unwired: 14 in]
          }
          frame "UI: Front Panel State" {
            # "Argument"
            # "Set Front Panel Open or Closed\n(Usage: \"UI: Front Panel State >> Open|Close\")"
            n88 = Unbundle By Name(w231) -> ("Core.Current VI Reference"=w230:refnum<vi>)
            n89 = disable-structure shown="Default" {
              disable-tunnel: w233 -> [w239 w262]
              disable-tunnel: [w238 w262] -> w232
              disable-tunnel: w230 -> [w237 _]
              disable-tunnel: w229 -> [w236 _]
              frame condition #0 (active) {
                n90 = case shown="\"Close\"" w236 {
                  tunnel: w239 -> [w243 w256]
                  tunnel: [w245 w257] -> w238
                  tunnel: w237 -> [w244 w254]
                  frame "Open", Default {
                    n91 = property class="VI"(reference=w244, error in=w243) -> (reference out=w241:refnum<vi>, error out=w242:errorcluster, "FP.State"=w240:T3)
                    n92 = case shown="Default" w240 {
                      tunnel: [w248 w251] -> w245
                      tunnel: w242 -> [w247 w251]
                      tunnel: w241 -> [w246 _]
                      frame "Closed" {
                        n93 = invoke class="VI" method="FP.Open"(reference=w246, error in=w247, "Activate"=TRUE, "State"=T3."Standard") -> (error out=w248:errorcluster)  [unwired: 1 in, 4 out]
                      }
                      frame Default {
                      }
                    }
                  }
                  frame "Close" {
                    n94 = property class="VI"(reference=w254, error in=w256) -> (reference out=w253:refnum<vi>, error out=w255:errorcluster, "FP.State"=w252:T3)
                    n95 = case shown="Default" w252 {
                      tunnel: [w258 w261] -> w257
                      tunnel: w255 -> [w258 w260]
                      tunnel: w253 -> [_ w259]
                      frame "Invalid", "Closed" {
                      }
                      frame Default {
                        n96 = invoke class="VI" method="FP.Close"(reference=w259, error in=w260) -> (error out=w261:errorcluster)  [unwired: 1 in, 2 out]
                      }
                    }
                  }
                }
              }
              frame condition #1 {
              }
            }
            n97 = call <vilib>:"Add State(s) to Queue__jki_lib_state_machine.vi"("State(s) in (\"\")"=w235) -> ("States Out"=w234:string)  [unwired: 14 in]
          }
          frame "UI: Wait" {
            n98 = Unbundle By Name(w265) -> ("Behavior"=w264:T7)
            n99 = case shown="\"Debug\"" w264 {
              tunnel: [u32 0 ("milliseconds to wait") u32 1000 ("milliseconds to wait")] -> w263
              frame "Normal", Default {
              }
              frame "Debug" {
              }
            }
            n100 = call <userlib>:"Wait (ms)__ogtk.vi"("error in (no error)"=w267, "milliseconds to wait"=w263) -> ("error out"=w266:errorcluster)  [unwired: 8 in, 1 out]
            n101 = call <vilib>:"Add State(s) to Queue__jki_lib_state_machine.vi"("State(s) in (\"\")"=w270) -> ("States Out"=w269:string)  [unwired: 14 in]
          }
          frame "---------- Macro ----------" {
            # "Do not put any code in this frame.\n(It is a separator no-op. You can make a copy of this frame to create a new Macro frame)"
            n102 = call <vilib>:"Add State(s) to Queue__jki_lib_state_machine.vi"("State(s) in (\"\")"=w277) -> ("States Out"=w276:string)  [unwired: 14 in]
          }
          frame "Macro: Initialize" {
            # "This needs to be called here before Data: Initialize\nto ensure that the correct argument is used"
            # "Initialization Macro\n(This is called once, when the VI starts)"
            n103 = call <userlib>:"Get Debug Mode.vi"("SMO"=w280) -> ("Behavior"=w278:T7)  [unwired: 8 in, 2 out]
            n104 = call-dynamic "Read Debug Mode.vi"("error in (no error)"=w285, "Instrument in"=w280) -> ("error out"=w284:errorcluster)  [unwired: 7 in, 2 out]
            n105 = case shown="\"Debug\"" w278 {
              tunnel: ["Close" "Open"] -> w279
              frame "Normal", Default {
              }
              frame "Debug" {
              }
            }
            n106 = Format Into String(format string="UI: Initialize\nUI: Front Panel State >> %s\nUI: Wait", initial string="", w279) -> (resulting string=w283:string)  [unwired: 1 in, 1 out]
            n107 = call <vilib>:"Add State(s) to Queue__jki_lib_state_machine.vi"("State(s) in Front (\"\")"="Data: Initialize\nInitialize Core Data\nEvents: Register", "State(s) in (\"\")"="Process: Sync", "State(s) at Back (\"\")"=w283) -> ("States Out"=w288:string)  [unwired: 12 in]
            n108 = call <vilib>:"Add State(s) to Queue__jki_lib_state_machine.vi"("State(s) in Front (\"\")"=w288, "State(s) in (\"\")"=w292) -> ("States Out"=w291:string)  [unwired: 13 in]
          }
          frame "Macro: Exit" {
            # "Exit Macro\n(This is called once, when the VI exits)"
            n109 = Unbundle By Name(w303) -> ("Behavior"=w297:T7, "Core.Close Panel on Exit?"=w308:bool)
            n110 = case shown="\"Debug\"" w297 {
              tunnel: ["Close" "Open"] -> w296
              frame "Normal", Default {
              }
              frame "Debug" {
              }
            }
            n111 = call <vilib>:"Build State String with Arguments__JKI_lib_State_Machine.vi"("Arguments (\"\")"=w296, "State"="UI: Front Panel State") -> ("State with Arguments"=w298:string)  [unwired: 4 in]
            n112 = Select(t=w298, s=w308, f="") -> (s? t:f=w306:string)
            n113 = call <vilib>:"Add State(s) to Queue__jki_lib_state_machine.vi"("State(s) in Front (\"\")"="Data: Cleanup\nEvents: Unregister", "State(s) in (\"\")"="Process: Sync", "State(s) at Back (\"\")"="Exit") -> ("States Out"=w300:string)  [unwired: 12 in]
            n114 = call <vilib>:"Add State(s) to Queue__jki_lib_state_machine.vi"("State(s) in (\"\")"=w306, "State(s) at Back (\"\")"=w300) -> ("States Out"=w305:string)  [unwired: 13 in]
            n115 = call <vilib>:"Add State(s) to Queue__jki_lib_state_machine.vi"("State(s) in Front (\"\")"=w305, "State(s) in (\"\")"=w311) -> ("States Out"=w310:string)  [unwired: 13 in]
          }
          frame "Macro: Post Error Handling" {
            # "Clear Last Error?"
            n116 = Unbundle By Name(w320) -> ("Core.Last Error.remaining states"=w322:string, "Core.Shutdown?"=w323:bool)
            n117 = Unbundle By Name(w320) -> ("Core.Last Error.error"=w315:errorcluster)
            n118 = case shown="False" FALSE {
              tunnel: w315 -> [w326 _]
              tunnel: [w326 _] -> w314
              frame False {
              }
              frame True {
              }
            }
            n119 = case shown="True" w323 {
              tunnel: w322 -> [w327 w329]
              tunnel: [w327 w328] -> w319
              frame False {
                # "These are the remaining states (at the moment the error occured). States can be altered according to business logic."
                # "NOT SHUTTING DOWN"
              }
              frame True {
                # "Developer can decide to alter the states but should be aware that during the shutdown process, there are certain states that must be run for the SMO to properly shut itself (and this process) down. As such, one can add states to perform additional clean-ups, but should append the remaining state to be executed."
                # "SHUTTING DOWN"
                n120 = call <vilib>:"Add State(s) to Queue__jki_lib_state_machine.vi"("State(s) in (\"\")"=w329) -> ("States Out"=w328:string)  [unwired: 14 in]
              }
            }
            n121 = Bundle By Name(cluster=w320, "Core.Last Error.error"=w314) -> (w321:T8)
            n122 = call <vilib>:"Add State(s) to Queue__jki_lib_state_machine.vi"("State(s) in Front (\"\")"=w319, "State(s) in (\"\")"=w317) -> ("States Out"=w318:string)  [unwired: 13 in]
          }
          frame "---------- Process ----------" {
            # "Template Separator\n(You can make a copy of, or modify, this frame)"
            n123 = call <vilib>:"Add State(s) to Queue__jki_lib_state_machine.vi"("State(s) in (\"\")"=w334) -> ("States Out"=w333:string)  [unwired: 14 in]
          }
          frame "Process: Sync" {
            n124 = Unbundle By Name(w342) -> ("SelfRef"=w338:refnum<class "Instrument.lvclass">)
            n125 = call <vilib>:"WaitOnProcessSync.vi"("error in (no error)"=w337, "SMO"=w338) -> ("error out"=w336:errorcluster, "Don't run?"=w341:bool)  [unwired: 7 in, 1 out]
            n126 = Select(t="Data: Cleanup\nEvents: Unregister\nExit", s=w341, f="") -> (s? t:f=w335:string)
            n127 = call <vilib>:"Add State(s) to Queue__jki_lib_state_machine.vi"("State(s) in Front (\"\")"=w335, "State(s) in (\"\")"=w345) -> ("States Out"=w344:string)  [unwired: 13 in]
          }
          frame "Process: SelfTerminate" {
            # "Template Separator\n(You can make a copy of, or modify, this frame)"
            n128 = Unbundle By Name(w349) -> ("SelfRef"=w351:refnum<class "Instrument.lvclass">)
            n129 = call <vilib>:"SelfTerminate.vi"("error in (no error)"=w347, "SMO in"=w351) -> ("error out"=w346:errorcluster, "SMO out"=w350:refnum<class "Instrument.lvclass">)  [unwired: 8 in]
            n130 = Bundle By Name(cluster=w349, "SelfRef"=w350) -> (w348:T8)
            n131 = call <vilib>:"Add State(s) to Queue__jki_lib_state_machine.vi"("State(s) in (\"\")"=w354) -> ("States Out"=w353:string)  [unwired: 14 in]
          }
          frame "---------- Events ----------" {
            # "Template Separator\n(You can make a copy of, or modify, this frame)"
            n132 = call <vilib>:"Add State(s) to Queue__jki_lib_state_machine.vi"("State(s) in (\"\")"=w359) -> ("States Out"=w358:string)  [unwired: 14 in]
          }
          frame "Events: Register" {
            n133 = Unbundle By Name(w388) -> ("SelfRef"=w383:refnum<class "Instrument.lvclass">, "Dependencies.Remote-Control"=w382:refnum<class "RemoteControl.lvclass">, "Dependencies.DB-Logger"=w377:refnum<class "Logger.PGSQL.lvclass">, "Dependencies.Error-Logger"=w378:refnum<class "Logger.Error.lvclass">)
            n134 = call <vilib>:"GetProtectedEvents.vi"("SMO"=w383) -> ("error out"=w385:errorcluster, "SMO Protected Events"=w373:T11, "SMO out"=w376:refnum<class "Instrument.lvclass">)  [unwired: 8 in]
            n135 = call "Instrument.GetPrivateEvents.vi"("Instrument"=w376) -> ("error out"=w372:errorcluster, "Instrument Private Events"=w370:T12)  [unwired: 8 in, 1 out]
            n136 = call <userlib>:"RemoteControl.GetPublicEvents.vi"("RemoteControl"=w382) -> ("error out"=w371:errorcluster, "RC Public Events"=w369:T13, "RemoteControl out"=w375:refnum<class "RemoteControl.lvclass">)  [unwired: 8 in]
            n137 = call <vilib>:"GetPublicEvents.vi"("SMO"=w375) -> ("error out"=w381:errorcluster, "Public Events"=w368:T14)  [unwired: 8 in, 1 out]
            n138 = call <vilib>:"GetPublicEvents.vi"("SMO"=w377) -> ("error out"=w380:errorcluster, "Public Events"=w366:T14)  [unwired: 8 in, 1 out]
            n139 = call <vilib>:"GetPublicEvents.vi"("SMO"=w378) -> ("error out"=w379:errorcluster, "Public Events"=w363:T14)  [unwired: 8 in, 1 out]
            n140 = call "Rename RC SMO Private Events.vi"("error in (no error)"=w381, "Public Events"=w368) -> ("error out"=w360:errorcluster, "RC SMO Public Events"=w367:T14)  [unwired: 8 in]
            n141 = call "Rename PGSQL SMO Private Events.vi"("error in (no error)"=w380, "Public Events"=w366) -> ("error out"=w361:errorcluster, "PGSQL SMO Public Events"=w365:T14)  [unwired: 8 in]
            n142 = call "Rename Error SMO Private Events.vi"("error in (no error)"=w379, "Public Events"=w363) -> ("error out"=w364:errorcluster, "Error SMO Public Events"=w362:T14)  [unwired: 8 in]
            n143 = register-events(w373, w370, w369, w367, w365, w362) -> (reference out=w387:refnum<event-registration>, error out=w374:errorcluster)  [unwired: 2 in]
            n144 = Merge Errors(w374, w360, w361, w364, w371, w372, w385, w384) -> (w386:errorcluster)
            n145 = call <vilib>:"Add State(s) to Queue__jki_lib_state_machine.vi"("State(s) in (\"\")"=w390) -> ("States Out"=w389:string)  [unwired: 14 in]
          }
          frame "Events: Unregister" {
            n146 = Unregister For Events(event registration refnum=w393, error in=w392) -> (error out=w391:errorcluster)
            n147 = call <vilib>:"Clear Errors.vi"("error in (no error)"=w391) -> ()  [unwired: 5 in, 2 out]
            n148 = call <vilib>:"Add State(s) to Queue__jki_lib_state_machine.vi"("State(s) in (\"\")"=w396) -> ("States Out"=w395:string)  [unwired: 14 in]
          }
          frame "---------- Instrument ----------" {
            n149 = call <vilib>:"Add State(s) to Queue__jki_lib_state_machine.vi"("State(s) in (\"\")"=w401) -> ("States Out"=w400:string)  [unwired: 14 in]
          }
          frame "Instrument: Handle Command" {
            # "parse and handle incoming commands\n- respond with data on hand\n- forward message to child instrument...etc"
            n150 = Unbundle By Name(w417) -> ("Dependencies.Remote-Control"=w421:refnum<class "RemoteControl.lvclass">, "SelfRef"=w418:refnum<class "Instrument.lvclass">, "Message.Command"=w402:string, "Message.Data"=w415:variant, "Message.ID"=w419:string)
            n151 = Format Into String(format string="%s Command:  %s", w404, w402) -> (resulting string=→"Command":string)  [unwired: 2 in, 1 out]
            n152 = call-dynamic "Handle Command.vi"("error in (no error)"=w420, "params in"=w415, "command"=w402, "Instrument in"=w418) -> ("error out"=w408:errorcluster, "processed data"=w411:variant, "command out"=w410:string, "Instrument out"=w407:refnum<class "Instrument.lvclass">)  [unwired: 4 in]
            n153 = Empty String/Path?(string/path=w410) -> (empty?=w414:bool)
            n154 = Empty String/Path?(string/path=w411) -> (empty?=w413:bool)
            n155 = And(x=w414, y=w413) -> (x .and. y?=w412:bool)
            n156 = case shown="False" w412 {
              tunnel: w421 -> [w433 _]
              tunnel: w408 -> [w429 w451]
              tunnel: w411 -> [w431 _]
              tunnel: w419 -> [w432 _]
              tunnel: [w428 w451] -> w409
              tunnel: w410 -> [w430 _]
              tunnel: w404 -> [w427 _]
              tunnel: w407 -> [w426 w450]
              tunnel: [w425 w450] -> w406
              frame False {
                # "command respond"
                n157 = case shown="\"Remote\"" w427 {
                  tunnel: w433 -> [_ w449]
                  tunnel: w432 -> [w435 w448]
                  tunnel: w431 -> [w437 w442]
                  tunnel: w430 -> [w438 w441]
                  tunnel: w429 -> [w436 w447]
                  tunnel: [w434 w446] -> w428
                  tunnel: w426 -> [w440 w443]
                  tunnel: [w439 w443] -> w425
                  frame "Local", Default {
                    n158 = call "Instrument.sendMessageFromProcess.vi"("ID"=w435, "error in (no error)"=w436, "Data"=w437, "Command"=w438, "Instrument"=w440) -> ("error out"=w434:errorcluster, "Instrument out"=w439:refnum<class "Instrument.lvclass">)  [unwired: 5 in]
                  }
                  frame "Remote" {
                    n159 = Bundle By Name(cluster=T4 {"Command"="", "Data"=variant(string ""), "ID"=""} ("Message"), "Command"=w441, "Data"=w442, "ID"=w448) -> (w444:T4)
                    n160 = call <userlib>:"RemoteControl.SendMessageToProcess.vi"("error in (no error)"=w447, "Message"=w444, "RemoteControl"=w449) -> ("error out"=w446:errorcluster)  [unwired: 7 in, 1 out]
                  }
                }
              }
              frame True {
              }
            }
            n161 = Bundle By Name(cluster=w417, "SelfRef"=w406) -> (w416:T8)
            n162 = call <vilib>:"Add State(s) to Queue__jki_lib_state_machine.vi"("State(s) in (\"\")"=w424) -> ("States Out"=w423:string)  [unwired: 14 in]
          }
          frame "Instrument: Log Data" {
            # "send event to PGSQL process"
            n163 = Unbundle By Name(w455) -> ("Dependencies.DB-Logger"=w458:refnum<class "Logger.PGSQL.lvclass">, "SelfRef"=w454:refnum<class "Instrument.lvclass">)
            n164 = Unbundle By Name(w454) -> ("path"=w453:string, "Data"=w452:variant)
            n165 = call <userlib>:"Logger.PGSQL.WriteVariable.vi"("error in (no error)"=w457, "Data"=w452, "Address"=w453, "Logger"=w458) -> ("error out"=w456:errorcluster)  [unwired: 6 in, 1 out]
            n166 = call <vilib>:"Add State(s) to Queue__jki_lib_state_machine.vi"("State(s) in (\"\")"=w461) -> ("States Out"=w460:string)  [unwired: 14 in]
          }
        }
      }
    }
    frame Error {
    }
  }
  n167 = call-parent "Process.vi"("error in"=w5, "SMO"=w4) -> ("error out"=w2:errorcluster, "SMO out"=→"Instrument out":refnum<class "Instrument.lvclass">)  [unwired: 8 in]
  n168 = Merge Errors(w2, w1) -> (→"error out":errorcluster)
